vi "File Read Options.vi"(1 "NameIn":string, 2 "DirIn":path, 5 "ErrorIn (no error)":errorcluster, 6 "File Read Mode":enum16{"Never", "List", "Ask"}(ring), 7 "ErrMsgOff":bool) -> (11 "FileList":string[](array[string]), 13 "ListLen":i32, 14 "PathOut":path, 15 "NameOut":string, 16 "DirOut":path, 17 "DirErr":bool, 18 "NameErr":bool, 19 "ErrorOut":errorcluster)   [LabVIEW 2013]
doc: "Modified 2/2001 to handle \"Canceled\" operation differently (error 43 is returned vs 8)\n\nThis vi can be used to provide directory and file information to file read vi's (use the File Write Options.vi for write-only operations or the File Delete Options.vi for deleting files). In particular it can be used to indicate whether the directory and file exist, to prompt for a filename if one is not supplied, and to provide a list of files in a directory which match a pattern. It does no actual file I/O other than verifying directories or files, or listing files. Although it is generally embedded in another vi, it can be used alone if only file information is required.\n\n In particular this vi performs a single file permission function concerned with reading an existing file or listing files in a directory. This function has the three attributes of Never, List, and Ask'. See \"VI OPERATION\" below for information on each mode.\n\nThis vi signals success or failure using two output error Booleans: DirErr and NameErr. If either is TRUE then subsequent reads from the file should be suppressed because either the directory or file does not exist or a related file I/O error occurred. It should be noted that error messages from canceled operations are suppressed.\n\nINPUT PARAMETERS\n------------------------------------\nDirIn - the drive letter and directory of the desired file such as \"C:\\\" or \"F:\\Master\\Source\"; the default is \"<not-a-path>\";\n\nNameIn - the filename and extension of the desired file such as \"Master.cfg\", or the pattern to use for listing files; the default is a null string;\n\nFile Read Mode - this enumerated control determines the function the vi performs and the manner in which it operates (see \"VI OPERATION\" below); the default is \"Never\". The \"Never\" mode is used to retrieve a file which should already exist; if it does not, an error is returned. The \"List\" mode is used to return a list of files that match the specified pattern in the specified directory; if the directory does not exist, an error is returned. The \"Ask\" mode is used to retrieve a file specified at runtine using a file dialog box.\n\nErrMsgOff - a Boolean (default = FALSE) which if TRUE will suppress the presentation of error messages (the Error Out cluster is still valid);\n\nErrorIn - a standard LabVIEW error cluster; if the Error In cluster contains an existing error, this vi performs no function.\n\n\nOUTPUT PARAMETERS\n----------------------------------------\nDirOut - the drive and directory to be used if no directory error; otherwise \"<not-a-path>\";\n\nNameOut - the filename and extension to be used if the file exists; otherwise a null string;\n\nPathOut - the combination of DirOut and NameOut including \"<not-a-path>\";\n\nFileList - a list (array) of the files found in directory DirIn which match the pattern specified by NameIn (valid only if the File Read Mode is \"List\"); if NameIn is empty, then the pattern \"*.*\" is used. If the File Read Mode is anything other than \"List\", then FileList is an empty array;\n\nListLen - the number of entries in the FileList array (0 if File Read Mode <> \"List\");\n\nDirErr - TRUE if unable to locate the specified directory; FALSE otherwise;\n\nNameErr - TRUE if unable to locate the specified file in directory DirOut or if DirErr is TRUE; FALSE otherwise;\n\nErrorOut - a standard LabVIEW error cluster. If the Error In cluster contained a previous error, then Error Out is Error In; otherwise Error Out is equal to the first error that occurs during execution (hopefully \"not-an-error\").\n\n\nVI OPERATION\n-------------------------\nOperation on the input proceeds in the sequence in which the processing states are listed below. The first detected fatal error causes an immediated jump to state \"Bad Done\"; any further processing is immediately terminated.\n\nFile Read Start - processing always starts here where the existence of the directory and file are separately determined. Based on this determination and on the value of control File Read Mode, a jump is either made to one of the other five states.\n\nNever Ask - this state (File Read Mode = \"Never\") results from the detection of a nonexistent file and the refused permission to ask for the file. A file permission error 8 is returned, PathOut is \"<not-a-path>\", DirOut is equal to DirIn if that directory exists, NameOut is NameIn, either DirErr or NameErr is TRUE depending on whether DirIn existed, FileList is empty, and FileLen is zero;\n\nList Files - when File Read Mode = \"List\", this vi returns a list of files which match the pattern specifed by NameIn such as \"*.*\" or \"*.txt\". The directory specified by DirIn must be a valid directory or an error is returned. If NameIn is empty, then the patten \"*.*\" is used. If all goes well, the list of files is returned in the string array FileList, the number of elements in ListLen, PathOut is <not-a-path>, DirOut is DirIn, NameOut is a null string, and both DirErr and NameErr are FALSE; note that error code 43 is returned but the \"Cancel\" message is suppressed. If any error is detected, FileList is empty and ListLen is zero, PathOut is <not-a-path>, DirOut are equal to DirIn, NameOut is a null string, DirErr is FALSE, and NameErr is TRUE;\n\nAlways Ask - when File Read Mode = \"Ask\" and the file as specified by DirIn and Namein does not already exist, then the user is presented with a file dialog box which can be used to choose a file to read. If successful, then PathOut is the path used, DirOut contains the name of the directory in which the file exists, NameOut contains the name of the selected file, DirErr and NameErr are both FALSE. If the user canceled the operation, then DirOut is equal to \"<not-a-path>\", NameOut is null, DirErr is TRUE or FALSE depending on whether DirIn exists, and NameErr is TRUE. If the file already exists, then no dialog box is presented, DirOut is set equal to DirIn, NameOut is NameIn, PathOut is DirIn concatenated with NameIn, and DirErr and NameErr are both FALSE."
panel:
  out "CurState":T1(ring)
  # "Err 1 - no Dir supplied\nErr 6 - generic file I/O\nErr 7 - file not found\nErr 8 - file permission\nErr 10 - duplicate path\nErr 43 - user canceled"
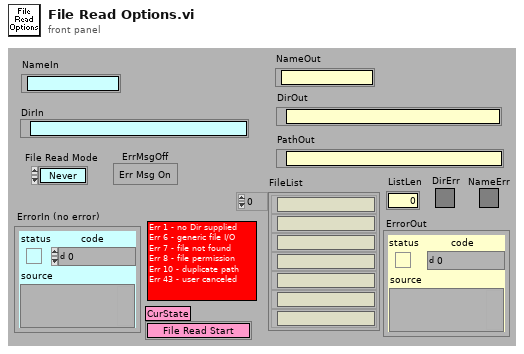
[diagram p1: front panel]
types:
  T1 = enum16{"File Read Start", "Never Ask", "List Files", "Always Ask", "Bad Done", "Good Done"}
  T2 = enum32{"existing file", "new file", "new or existing file", "existing dir", "new dir", "new or existing dir", "existing file (use LLBs)", "new file (use LLBs)", "new or existing file (use LLBs)", "new or existing file or directory (use LLBs)"}
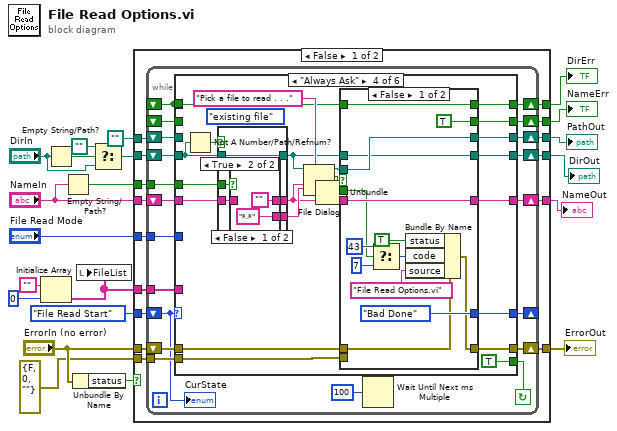
[diagram p0: block diagram]
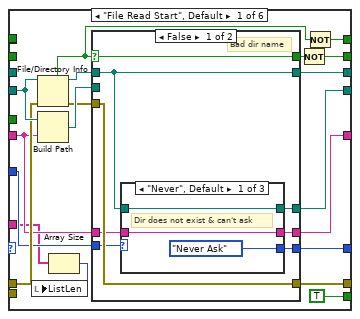
[diagram p2: hidden frame]
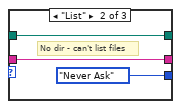
[diagram p3: hidden frame]
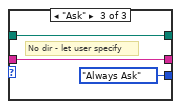
[diagram p4: hidden frame]
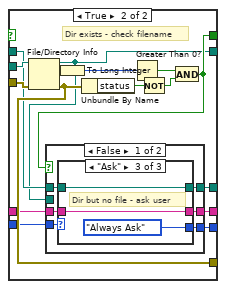
[diagram p5: hidden frame]
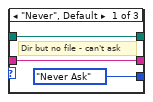
[diagram p6: hidden frame]
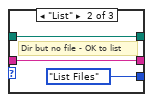
[diagram p7: hidden frame]
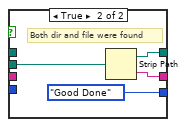
[diagram p8: hidden frame]
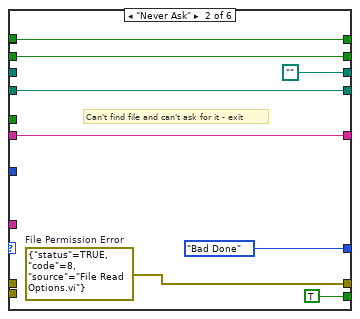
[diagram p9: hidden frame]
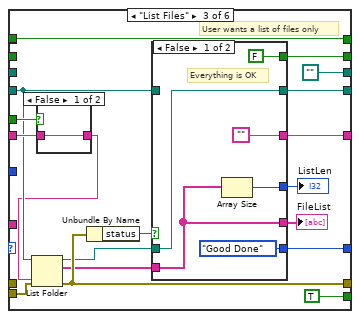
[diagram p10: hidden frame]
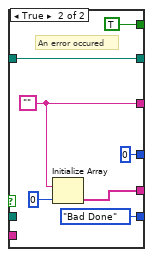
[diagram p11: hidden frame]
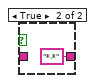
[diagram p12: hidden frame]
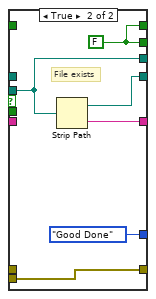
[diagram p13: hidden frame]
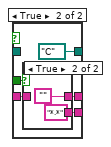
[diagram p15: hidden frame]
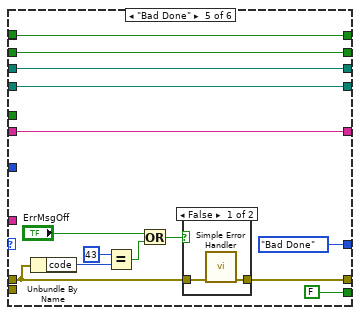
[diagram p17: hidden frame]
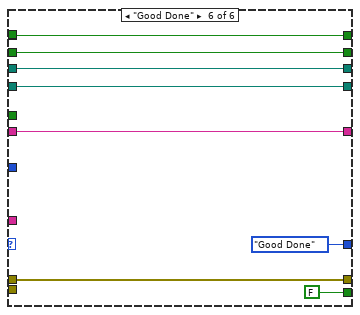
[diagram p19: hidden frame]
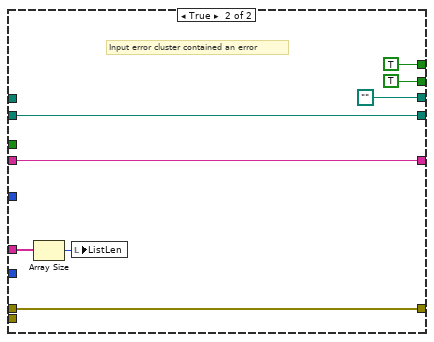
[diagram p20: hidden frame]
diagram:
  n1 = Initialize Array("", 0 ("Dimension Size")) -> (w1:string[])
  n2 = Empty String/Path?(string/path="DirIn") -> (empty?=w20:bool)
  n3 = Empty String/Path?(string/path="NameIn") -> (empty?=w4:bool)
  n4 = Unbundle By Name("ErrorIn (no error)") -> ("status"=w7:bool)
  n5 = local write "FileList"(w1) -> ()
  n6 = Select(t=path "", s=w20, f="DirIn") -> (s? t:f=w17:path)
  n7 = case shown="False" w7 {
    tunnel: T1."File Read Start" -> [w36 _]
    tunnel: w17 -> [w35 w256]
    tunnel: "NameIn" -> [w34 w255]
    tunnel: path "" -> [w33 _]
    tunnel: "ErrorIn (no error)" -> [w32 w258]
    tunnel: [w31 TRUE] -> w14
    tunnel: [w30 TRUE] -> w13
    tunnel: [w29 path ""] -> w12
    tunnel: [w28 w256] -> w11
    tunnel: [w27 w255] -> w10
    tunnel: [w26 w258] -> w9
    tunnel: "File Read Mode" -> [w25 _]
    tunnel: errorcluster {"status"=FALSE, "code"=0, "source"=""} ("ErrorOut") -> [w24 _]
    tunnel: w4 -> [w23 _]
    tunnel: w1 -> [w22 w254]
    frame False {
      n8 = while {
        tunnel: w22 -> [w37]
        tunnel: w23 -> [w40]
        tunnel: w24 -> [w42]
        tunnel: w25 -> [w45]
        shift-left: w32 -> [w52]
        shift-right: [w48] -> w26
        shift-left: _ -> [w39]
        shift-right: [w55] -> w31
        shift-left: _ -> [w46]
        shift-right: [w38] -> w30
        shift-left: w33 -> [w43]
        shift-right: [w51] -> w29
        shift-left: w34 -> [w53]
        shift-right: [w49] -> w27
        shift-left: w35 -> [w54]
        shift-right: [w50] -> w28
        shift-left: w36 -> [w41]
        shift-right: [w47] -> _
        stop <- w44 continue-if-true
        n9 = case shown="\"Always Ask\"" w41 {
          tunnel: [w72 w135 w141 w173 w241 w252] -> w55
          tunnel: w54 -> [w70 w128 w140 w188 w238 w249]
          tunnel: w53 -> [w59 w133 w150 w185 w237 w248]
          tunnel: w52 -> [w69 _ _ w176 w233 w246]
          tunnel: [w64 path "" path "" w181 w239 w250] -> w51
          tunnel: [w61 w128 w143 w180 w238 w249] -> w50
          tunnel: [w60 w133 w144 w179 w237 w248] -> w49
          tunnel: [w68 w130 w149 w177 w234 w246] -> w48
          tunnel: [w62 T1."Bad Done" w147 w183 T1."Bad Done" T1."Good Done"] -> w47
          tunnel: w39 -> [_ w135 _ w172 w241 w252]
          tunnel: w46 -> [_ w134 _ _ w240 w251]
          tunnel: w45 -> [w63 _ _ _ _ _]
          tunnel: [TRUE TRUE TRUE TRUE FALSE FALSE] -> w44
          tunnel: w43 -> [_ _ _ _ w239 w250]
          tunnel: w42 -> [_ _ w152 w170 _ _]
          tunnel: w40 -> [_ _ w151 w186 _ _]
          tunnel: w39 -> [_ _ w141 _ _ _]
          tunnel: [w71 w134 w142 w178 w240 w251] -> w38
          tunnel: w37 -> [w58 _ _ _ _ _]
          frame "File Read Start", Default {
            n10 = File/Directory Info(path=w70, error in=w69) -> (path out=w73:path, directory=w66:bool, error out=w74:errorcluster)  [unwired: 4 out]
            n11 = Build Path(base path=w70, name or relative path=w59) -> (appended path=w75:path)
            n12 = Array Size(array=w58) -> (size(s)=w57:i32)
            n13 = local write "ListLen"(w57) -> ()
            n14 = case shown="False" w66 {
              selector: w66 -> [w82 _]
              tunnel: w75 -> [_ w108]
              tunnel: w74 -> [w83 w107]
              tunnel: [w83 w105] -> w68
              tunnel: [w82 w99] -> w65
              tunnel: w73 -> [w78 w98]
              tunnel: [w78 w94] -> w64
              tunnel: w63 -> [w81 w100]
              tunnel: [w80 w101] -> w62
              tunnel: [w79 w97] -> w61
              tunnel: [w76 w96] -> w60
              tunnel: w59 -> [w77 w95]
              frame False {
                # "Bad dir name"
                n15 = case shown="\"Never\", Default" w81 {
                  tunnel: [T1."Never Ask" T1."Never Ask" T1."Always Ask"] -> w80
                  tunnel: [w85 w89 w92] -> w79
                  tunnel: [w86 w88 w91] -> w76
                  tunnel: w77 -> [w86 w88 w91]
                  tunnel: w78 -> [w85 w89 w92]
                  frame "Never", Default {
                    # "Dir does not exist & can't ask"
                  }
                  frame "List" {
                    # "No dir - can't list files"
                  }
                  frame "Ask" {
                    # "No dir - let user specify"
                  }
                }
              }
              frame True {
                # "Dir exists - check filename"
                n16 = File/Directory Info(path=w108, error in=w107) -> (path out=w94:path, size=w93:i64, error out=w105:errorcluster)  [unwired: 4 out]
                n17 = To Long Integer(number=w93) -> (32bit integer=w106:i32)
                n18 = Unbundle By Name(w105) -> ("status"=w103:bool)
                n19 = Greater Than 0?(x=w106) -> (x > 0?=w104:bool)
                n20 = Not(x=w103) -> (.not. x?=w102:bool)
                n21 = And(x=w104, y=w102) -> (x .and. y?=w99:bool)
                n22 = case shown="False" w99 {
                  tunnel: w100 -> [w114 _]
                  tunnel: [w113 T1."Good Done"] -> w101
                  tunnel: [w111 w127] -> w97
                  tunnel: [w110 w126] -> w96
                  tunnel: w94 -> [_ w125]
                  tunnel: w98 -> [w112 _]
                  tunnel: w95 -> [w109 _]
                  frame False {
                    n23 = case shown="\"Ask\"" w114 {
                      tunnel: [T1."Never Ask" T1."List Files" T1."Always Ask"] -> w113
                      tunnel: w112 -> [w117 w119 w123]
                      tunnel: [w117 w119 w123] -> w111
                      tunnel: [w116 w120 w122] -> w110
                      tunnel: w109 -> [w116 w120 w122]
                      frame "Never", Default {
                        # "Dir but no file - can't ask"
                      }
                      frame "List" {
                        # "Dir but no file - OK to list"
                      }
                      frame "Ask" {
                        # "Dir but no file - ask user"
                      }
                    }
                  }
                  frame True {
                    # "Both dir and file were found"
                    n24 = Strip Path(path=w125) -> (stripped path=w127:path, name=w126:string)
                  }
                }
              }
            }
            n25 = Not(x=w65) -> (.not. x?=w71:bool)
            n26 = Not(x=w66) -> (.not. x?=w72:bool)
          }
          frame "Never Ask" {
            w130 = errorcluster {"status"=TRUE, "code"=8, "source"="File Read Options.vi"}  # File Permission Error
            # "Can't find file and can't ask for it - exit"
          }
          frame "List Files" {
            # "User wants a list of files only"
            n27 = case shown="False" w151 {
              tunnel: w150 -> [w167 _]
              tunnel: [w167 "*.*" ("NameIn")] -> w139
              frame False {
              }
              frame True {
              }
            }
            n28 = List Folder(path=w140, pattern=w139, error in=w152) -> (path out=w146:path, filenames=w145:string[], error out=w149:errorcluster)  [unwired: 1 in, 1 out]
            n29 = Unbundle By Name(w149) -> ("status"=w148:bool)
            n30 = case shown="False" w148 {
              tunnel: [T1."Good Done" T1."Bad Done"] -> w147
              tunnel: w146 -> [w157 _]
              tunnel: w145 -> [w155 _]
              tunnel: ["" w163] -> w144
              tunnel: [w157 w164] -> w143
              tunnel: [FALSE TRUE] -> w142
              tunnel: w140 -> [_ w164]
              tunnel: [w156 0] -> w138
              tunnel: [w155 w161] -> w137
              frame False {
                # "Everything is OK"
                n31 = Array Size(array=w155) -> (size(s)=w156:i32)
              }
              frame True {
                w163 = ""
                # "An error occured"
                n32 = Initialize Array(w163, 0 ("Dimension Size")) -> (w161:string[])
              }
            }
            "ListLen" <- w138
            "FileList" <- w137
          }
          frame "Always Ask" {
            (unwired) T1."Bad Done"
            (unwired) T2."existing file" ("select mode (2)")
            n33 = Not A Number/Path/Refnum?(number/path/refnum=w188) -> (NaN/Path/Refnum?=w189:bool)
            n34 = case shown="False" w189 {
              tunnel: w188 -> [w216 _]
              tunnel: [w216 path "C:/" ("t")] -> w175
              tunnel: [w213 w221] -> w174
              tunnel: [w212 w220] -> w187
              tunnel: w186 -> [w215 w223]
              tunnel: w185 -> [w214 w222]
              frame False {
                n35 = case shown="True" w215 {
                  tunnel: w214 -> [w217 _]
                  tunnel: [w217 ""] -> w213
                  tunnel: [w217 "*.*" ("t")] -> w212
                  frame False {
                  }
                  frame True {
                  }
                }
              }
              frame True {
                n36 = case shown="True" w223 {
                  tunnel: w222 -> [w225 _]
                  tunnel: [w225 ""] -> w221
                  tunnel: [w225 "*.*"] -> w220
                  frame False {
                  }
                  frame True {
                  }
                }
              }
            }
            n37 = File Dialog(6:w187, 7:"Pick a file to read . . ." ("prompt"), 9:w174, 11:w175) -> (0:w169:errorcluster, 1:w171:bool, 2:w184:bool, 3:w182:path)  [unwired: 3 in]
            n38 = Unbundle(w169) -> ()  [unwired: 3 out]
            n39 = case shown="False" w184 {
              tunnel: [T1."Bad Done" T1."Good Done"] -> w183
              tunnel: w182 -> [w204 w210]
              tunnel: [w204 w210] -> w181
              tunnel: [w203 w209] -> w180
              tunnel: [w202 w208] -> w179
              tunnel: [TRUE w207] -> w178
              tunnel: [w199 w206] -> w177
              tunnel: w176 -> [w198 _]
              tunnel: w175 -> [w203 _]
              tunnel: w174 -> [w202 _]
              tunnel: [w200 w207] -> w173
              tunnel: w172 -> [w200 _]
              tunnel: w171 -> [w192 _]
              tunnel: w170 -> [_ w206]
              frame False {
                n40 = Select(t=43, s=w192, f=7 ("code")) -> (s? t:f=w195:i32)
                n41 = Bundle By Name(cluster=w198, "status"=TRUE ("Bundle Element"), "code"=w195, "source"="File Read Options.vi" ("Bundle Element")) -> (w199:errorcluster)
              }
              frame True {
                w207 = FALSE
                # "File exists"
                n42 = Strip Path(path=w210) -> (stripped path=w209:path, name=w208:string)
              }
            }
          }
          frame "Bad Done" {
            n43 = Unbundle By Name(w233) -> ("code"=w230:i32)
            n44 = Equal?(x=43, y=w230) -> (x = y?=w228:bool)
            n45 = Or(x="ErrMsgOff", y=w228) -> (x .or. y?=w232:bool)
            n46 = case shown="False" w232 {
              tunnel: [w242 w244] -> w234
              tunnel: w233 -> [w243 w244]
              frame False {
                n47 = call <vilib>:"Simple Error Handler.vi"("error in (no error)"=w243) -> ("error out"=w242:errorcluster)  [unwired: 4 in, 4 out]
              }
              frame True {
              }
            }
          }
          frame "Good Done" {
          }
        }
        n48 = Wait Until Next ms Multiple(millisecond multiple=u32 100) -> ()  [unwired: 1 out]
        "CurState" <- w41
      }
    }
    frame True {
      # "Input error cluster contained an error"
      n49 = Array Size(array=w254) -> (size(s)=w253:i32)
      n50 = local write "ListLen"(w253) -> ()
    }
  }
  "ErrorOut" <- w9
  "NameOut" <- w10
  "DirOut" <- w11
  "PathOut" <- w12
  "DirErr" <- w14
  "NameErr" <- w13
